vi "Write Angles.vi"(8 "error in (no error)":errorcluster, 10 "angles (rad)":dbl[](array[numeric]), 11 "Simu Delta Robot in":refnum<class "Simu Delta Robot.lvclass">) -> (0 "error out":errorcluster, 3 "Simu Delta Robot out":refnum<class "Simu Delta Robot.lvclass">)   [LabVIEW 2014, in "Simu Delta Robot.lvclass"]
uses:
  Simu Delta Robot.lvclass
  Simu Delta Robot.lvclass/Simu Delta Robot.ctl
  <instrlib>/Hitec HS400 Series/HAIOL/Hitec HS400 Series.lvclass
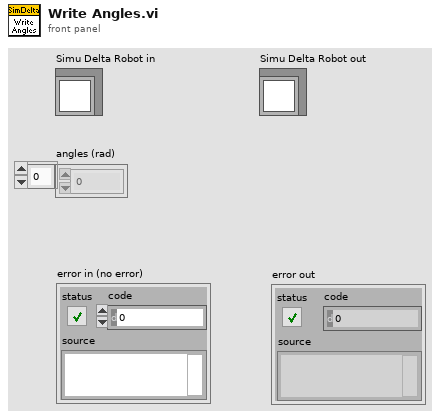
[diagram p1: front panel]
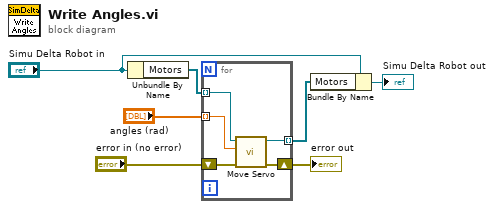
[diagram p0: block diagram]
diagram:
  n1 = Unbundle By Name("Simu Delta Robot in") -> ("Motors"=w7:refnum<class "Hitec HS400 Series.lvclass">[])
  n2 = for {
    tunnel: w7 -> [w12] mode=indexing
    shift-right: [w8] -> w2
    shift-left: "error in (no error)" -> [w11]
    tunnel: "angles (rad)" -> [w10] mode=indexing
    tunnel: [w9] -> w3 mode=indexing
    n3 = call-dynamic "Move Servo.vi"("error in (no error)"=w11, "CCW Position (0.0 rad)"=w10, "Hitec HS400 Series in"=w12) -> ("error out"=w8:errorcluster, "Hitec HS400 Series out"=w9:refnum<class "Hitec HS400 Series.lvclass">)  [unwired: 7 in]
  }
  "error out" <- w2
  n4 = Bundle By Name(cluster="Simu Delta Robot in", "Motors"=w3) -> (→"Simu Delta Robot out":refnum<class "Simu Delta Robot.lvclass">)
